vi "Get Serial Port List.vi"(8 "error in (no error)":errorcluster) -> (0 "error out":errorcluster, 1 "Port Names":string[](array[string]), 2 "#Ports":i32, 3 "VISA Name":string[](array[string]), 4 "Valid":bool[](array[boolean]))   [LabVIEW 2025]
doc: "Author: Scott Hannahs <sth@magnet.fsu.edu>\n\nThis software is licensed for use under the “MIT License\"\nCopyright (c) 2025 Scott Hannahs, sth@sth@magnet.sthnet.net\n\nPermission is hereby granted, free of charge, to any person obtaining a copy of this software and associated documentation files (the \"Software\"), to deal in the Software without restriction, including without limitation the rights to use, copy, modify, merge, publish, distribute, sublicense, and/or sell copies of the Software, and to permit persons to whom the Software is furnished to do so, subject to the following conditions: The above copyright notice and this permission notice shall be included in all copies or substantial portions of the Software.\n\nTHE SOFTWARE IS PROVIDED \"AS IS\", WITHOUT WARRANTY OF ANY KIND, EXPRESS OR IMPLIED, INCLUDING BUT NOT LIMITED TO THE WARRANTIES OF MERCHANTABILITY, FITNESS FOR A PARTICULAR PURPOSE AND NONINFRINGEMENT. IN NO EVENT SHALL THE AUTHORS OR COPYRIGHT HOLDERS BE LIABLE FOR ANY CLAIM, DAMAGES OR OTHER LIABILITY, WHETHER IN AN ACTION OF CONTRACT, TORT OR OTHERWISE, ARISING FROM, OUT OF OR IN CONNECTION WITH THE SOFTWARE OR THE USE OR OTHER DEALINGS IN THE SOFTWARE."
uses:
  <vilib>/Instr/_visa.llb/VISA Find Search Mode.ctl
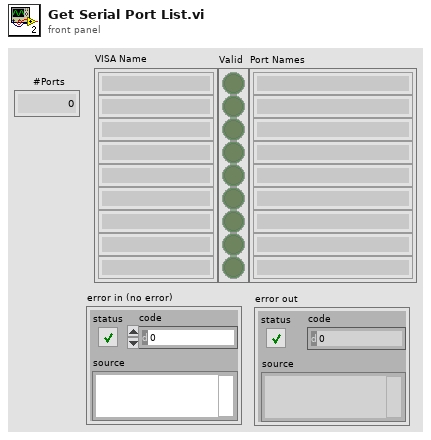
[diagram p1: front panel]
types:
  T1 = typedef "VISA Find Search Mode.ctl" = u32
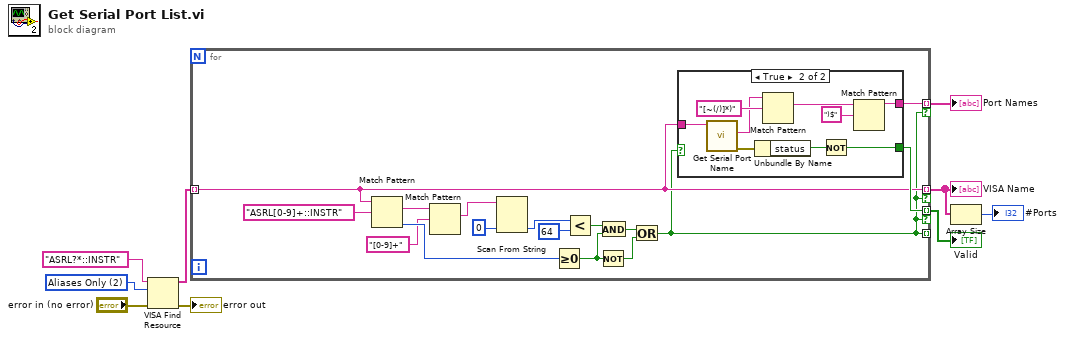
[diagram p0: block diagram]
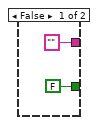
[diagram p2: hidden frame]
diagram:
  w3 = T1 2 items=["Canonical Names Only"=0, "Aliases Only"=2, "Include Matching Aliases"=3, "Include All Aliases"=4] ("Search Mode")
  n1 = VISA Find Resource(8:"error in (no error)", 10:w3, 11:"ASRL?*::INSTR" ("expression (\"\")")) -> (0:→"error out":errorcluster, 3:w1:string[])  [unwired: 1 out]
  n2 = for {
    tunnel: w1 -> [w11] mode=indexing
    tunnel: [w25] -> w7 mode=indexing if=w10
    tunnel: [w24] -> w6 mode=indexing if=w10
    tunnel: [w11] -> w8 mode=indexing if=w10
    tunnel: [w10] -> _ mode=indexing
    n3 = Match Pattern(string=w11, regular expression="ASRL[0-9]+::INSTR") -> (match substring=w13:string, offset past match=w20:i32)  [unwired: 1 in, 2 out]
    n4 = Match Pattern(string=w13, regular expression="[0-9]+") -> (match substring=w16:string)  [unwired: 1 in, 3 out]
    n5 = Scan From String(input string=w16, default 1=0 ("default value 1")) -> (output 1=w17:i32)  [unwired: 3 in, 3 out]
    n6 = Greater Or Equal To 0?(x=w20) -> (x >= 0?=w22:bool)
    n7 = Less?(x=w17, y=64) -> (x < y?=w19:bool)
    n8 = Not(x=w22) -> (.not. x?=w23:bool)
    n9 = And(x=w19, y=w22) -> (x .and. y?=w21:bool)
    n10 = Or(x=w21, y=w23) -> (x .or. y?=w10:bool)
    n11 = case shown="True" w10 {
      tunnel: [FALSE w35] -> w25
      tunnel: ["" ("Intf Inst Name") w31] -> w24
      tunnel: w11 -> [_ w30]
      frame False {
      }
      frame True {
        n12 = call "Get Serial Port Name.vi"("PS Communication Port In"=w30) -> ("Error Out"=w29:errorcluster, "Serial Port Name"=w28:string)  [unwired: 4 in, 1 out]
        n13 = Unbundle By Name(w29) -> ("status"=w36:bool)
        n14 = Match Pattern(string=w28, regular expression="[~(/)]*)") -> (match substring=w33:string)  [unwired: 1 in, 3 out]
        n15 = Not(x=w36) -> (.not. x?=w35:bool)
        n16 = Match Pattern(string=w33, regular expression=")$") -> (before substring=w31:string)  [unwired: 1 in, 3 out]
      }
    }
  }
  "VISA Name" <- w8
  "Valid" <- w7
  "Port Names" <- w6
  n17 = Array Size(array=w8) -> (size(s)=→"#Ports":i32)
